vi "Untitled 1.vi"() -> ()   [LabVIEW 2016]
uses:
  support/Message Queue/Message Queue.lvlib
  support/Message Queue/Enqueue Message (Single).vi
  controls/UI State.ctl
  Settings/Settings.lvlib
  support/User Event - Stop/User Event - Stop.lvlib
  <vilib>/Utility/error.llb/Error Cluster From Error Code.vi
  <vilib>/ErrorRing/Error Ring.xnode
panel:
  in  "PZTY+":bool
  in  "PZTX-":bool
  in  "PZTX+":bool
  in  "PZTY-":bool
  in  "PZTZ-":bool
  in  "PZTZ+":bool
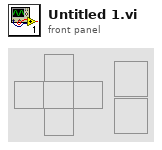
[diagram p1: front panel]
types:
  T1 = typedef "UI State.ctl" = enum16{"Idle", "Acquiring", "Acquiring Stopped", "Logging", "Logging Stopped"}
  T2 = typedef "Settings.lvlib/Settings.ctl" = cluster{"Hardware Configuration":T3, "Logging Configuration":T4, "PZT Configuration ":T5}
  T3 = typedef "Acquisition.lvlib/Hardware Configuration.ctl" = cluster{"DAQmx Input":tag, "Max Input":dbl, "Min Input":dbl, "Sample Rate":dbl, "DAQmx Task":refnum<k21>}
  T4 = typedef "Logging.lvlib/Logging Configuration.ctl" = cluster{"Log File Base Path":path, "TDMS File Reference":refnum<k34>, "Channel names":string[], "Author":string, "Description":string}
  T5 = typedef "PZT_Control.ctl" = cluster{"DAQmx Output":tag, "PZTX":dbl, "PZTY":dbl, "PZTZ":dbl, "Waveform Type":enum16{"Sine Wave", "Triangle Wave", "Square Wave", "Sawtooth Wave"}, "PZT_Amp":dbl, "PZT_Freq":dbl, "PZT_Phase":dbl}
  T6 = cluster{"Hardware Configuration":T3, "Logging Configuration":cluster{"Log File Base Path":path, "TDMS File Reference":refnum<k34>, "Channel names":string[], "Author":string, "Description":string}, "PZT Configuration ":T5}
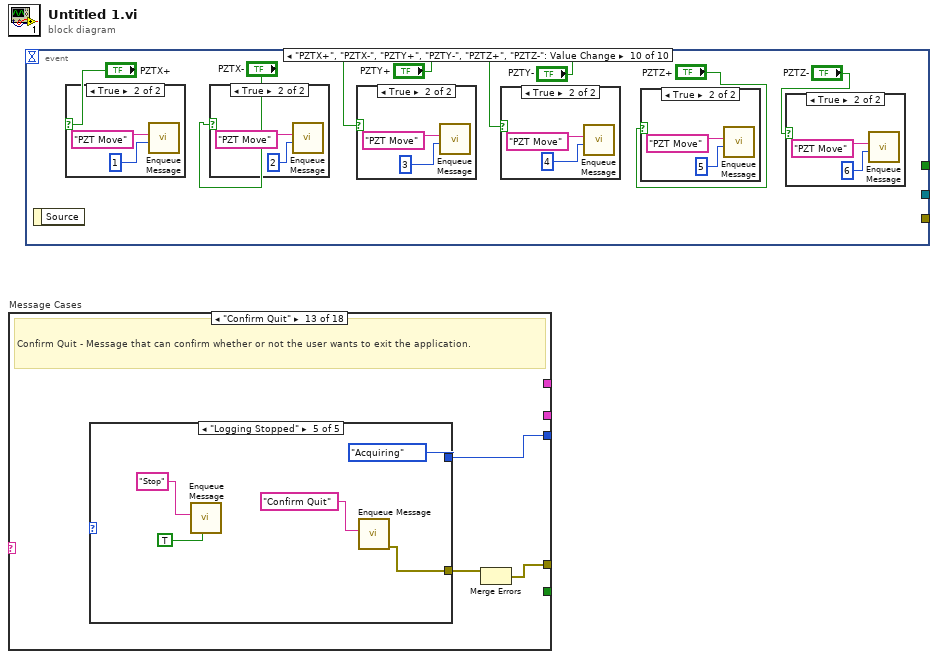
[diagram p0: block diagram]
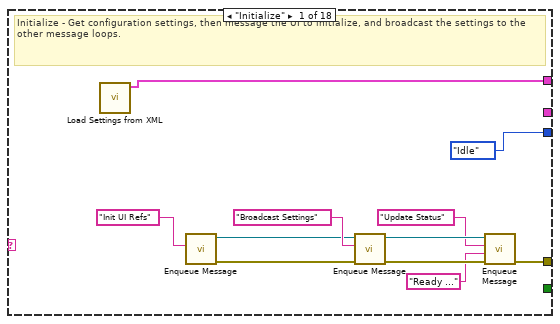
[diagram p2: hidden frame]
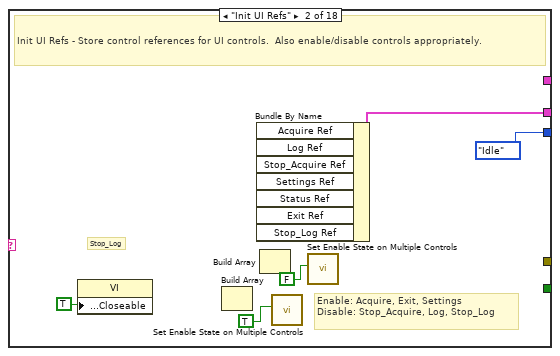
[diagram p3: hidden frame]
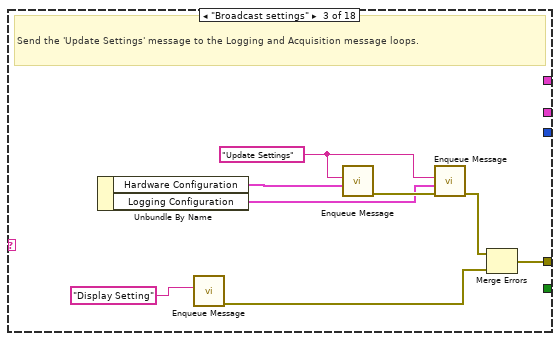
[diagram p4: hidden frame]
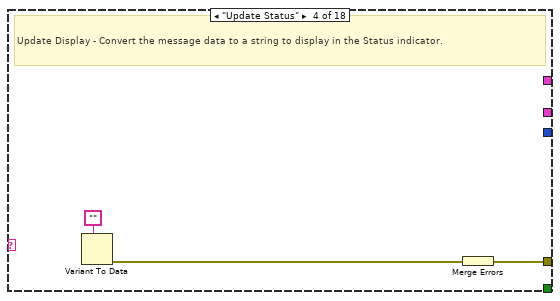
[diagram p5: hidden frame]
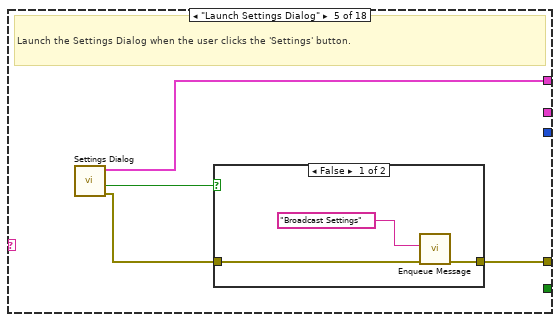
[diagram p6: hidden frame]
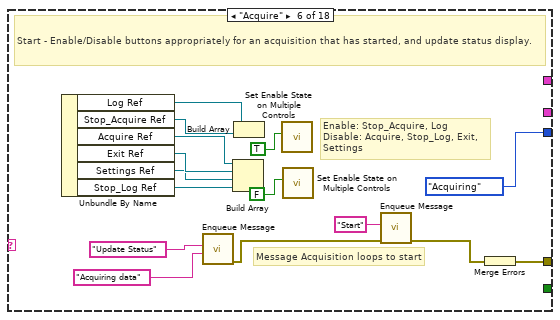
[diagram p8: hidden frame]
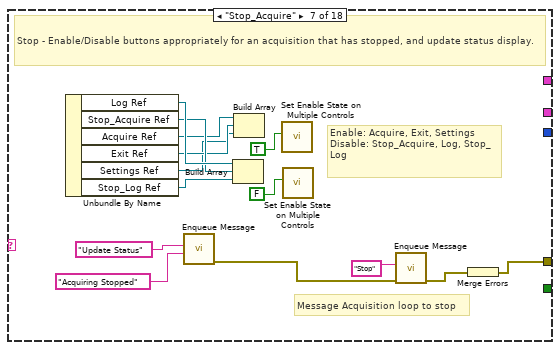
[diagram p9: hidden frame]
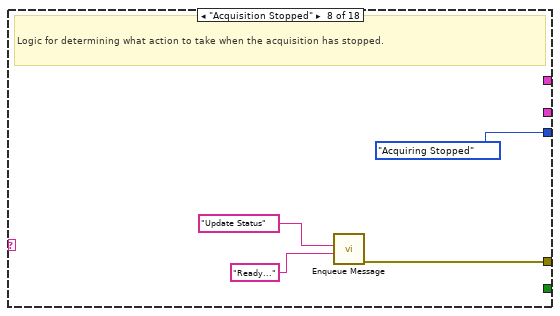
[diagram p10: hidden frame]
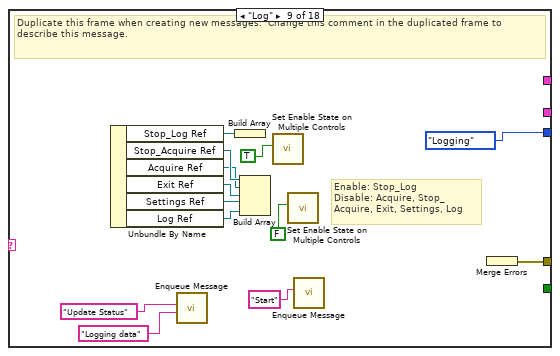
[diagram p11: hidden frame]
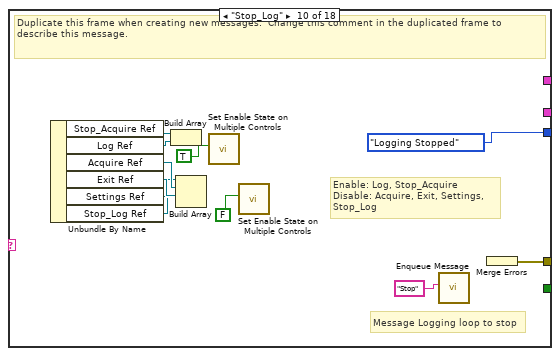
[diagram p12: hidden frame]
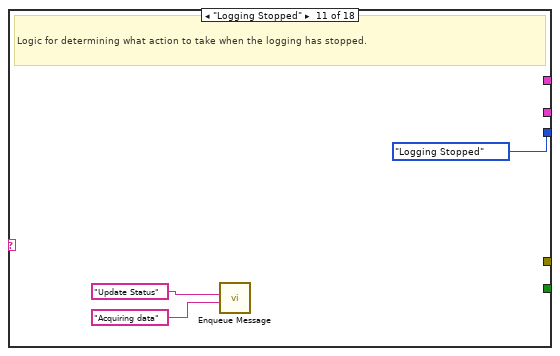
[diagram p13: hidden frame]
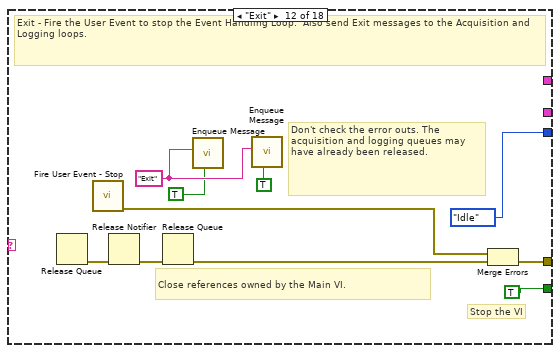
[diagram p14: hidden frame]
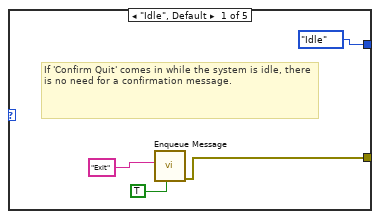
[diagram p15: hidden frame]
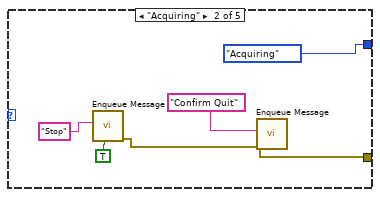
[diagram p16: hidden frame]
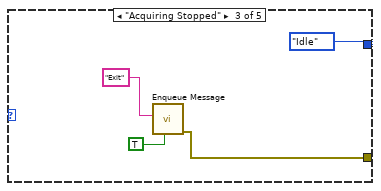
[diagram p17: hidden frame]
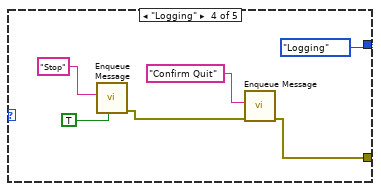
[diagram p18: hidden frame]
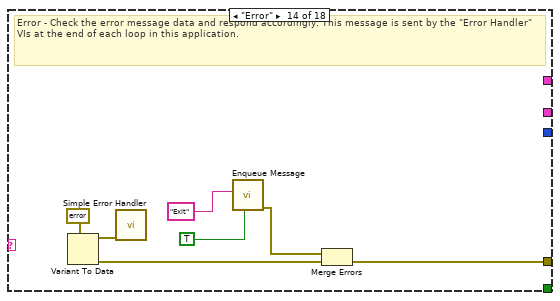
[diagram p19: hidden frame]
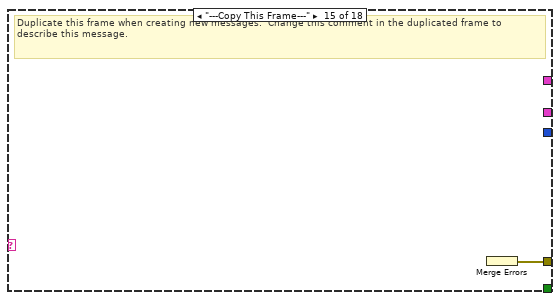
[diagram p20: hidden frame]
diagram:
  n1 = case "Message Cases" shown="\"Confirm Quit\"" {
    selector: _ -> [_ _ _ _ _ _ _ _ _ _ _ _ _ _ _ _ _ w145]
    tunnel: [w9 _ w24 w27 w29 w50 w64 w67 w81 w92 _ w104 w107 w134 w141 _ w144 w146] -> _
    tunnel: [_ _ _ _ _ _ _ _ _ _ _ TRUE _ _ _ _ _ _] -> _
    tunnel: [_ w16 _ _ _ _ _ _ _ _ _ _ _ _ _ _ _ _] -> _
    tunnel: [UI_State."Idle" ("UI State") UI_State."Idle" ("UI State") _ _ _ UI_State."Acquiring" ("UI State") _ UI_State."Acquiring Stopped" ("UI State") UI_State."Logging" ("UI State") UI_State."Logging Stopped" ("UI State") UI_State."Logging Stopped" ("UI State") UI_State."Idle" ("UI State") w108 _ _ _ _ _] -> _
    tunnel: [w1 _ _ _ w28 _ _ _ _ _ _ _ _ _ _ _ _ _] -> _
    frame "Initialize" {
      # "Initialize - Get configuration settings, then message the UI to initialize, and broadcast the settings to the other message loops."
      n2 = call "Load Settings from XML.vi"() -> ("Settings out"=w1:T2)  [unwired: 10 in, 1 out]
      n3 = call-poly "Enqueue Message.vi"("Message"="Init UI Refs") -> ("error out"=w3:errorcluster, "dup Message Queue"=w4:refnum<queue>)  [unwired: 9 in]
      n4 = call-poly "Enqueue Message.vi"("error in (no error)"=w3, "Message"="Broadcast Settings", "Message Queue"=w4) -> ("error out"=w11:errorcluster, "dup Message Queue"=w10:refnum<queue>)  [unwired: 7 in]
      n5 = call-poly "Enqueue Message.vi"("error in (no error)"=w11, "Message Data"="Ready ..." ("Ready..."), "Message"="Update Status", "Message Queue"=w10) -> ("error out"=w9:errorcluster)  [unwired: 6 in, 1 out]
    }
    frame "Init UI Refs" {
      # "Stop_Log"
      # "Enable: Acquire, Exit, Settings\nDisable: Stop_Acquire, Log, Stop_Log"
      # "Init UI Refs - Store control references for UI controls.  Also enable/disable controls appropriately."
      n6 = property class="VI"("Front Panel.Closeable"=TRUE ("Front Panel Window:Closeable")) -> ()  [unwired: 2 in, 2 out]
      n7 = Build Array() -> ()  [unwired: 3 in, 1 out]
      n8 = Bundle By Name() -> (w16:cluster{})  [unwired: 8 in]
      n9 = Build Array() -> ()  [unwired: 3 in, 1 out]
      n10 = call "Set Enable State on Multiple Controls.vi"("Enable?"=TRUE) -> ()  [unwired: 11 in]
      n11 = call "Set Enable State on Multiple Controls.vi"("Enable?"=FALSE) -> ()  [unwired: 11 in]
    }
    frame "Broadcast settings" {
      w19 = "Update Settings" ("Message")
      # "Send the 'Update Settings' message to the Logging and Acquisition message loops."
      n12 = Unbundle By Name() -> ("Hardware Configuration"=w22:T3, "Logging Configuration"=w21:T4)  [unwired: 1 in]
      n13 = call-poly "Enqueue Message.vi"("Message"="Display Setting") -> ("error out"=w17:errorcluster)  [unwired: 9 in, 1 out]
      n14 = call-poly "Enqueue Message.vi"("Message Data"=w22, "Message"=w19) -> ("error out"=w23:errorcluster)  [unwired: 8 in, 1 out]
      n15 = call-poly "Enqueue Message.vi"("error in (no error)"=w23, "Message Data"=w21, "Message"=w19) -> ("error out"=w20:errorcluster)  [unwired: 7 in, 1 out]
      n16 = Merge Errors(w20, w17) -> (w24:errorcluster)  [unwired: 1 in]
    }
    frame "Update Status" {
      # "Update Display - Convert the message data to a string to display in the Status indicator."
      n17 = Variant To Data(type="") -> (error out=w25:errorcluster)  [unwired: 2 in, 1 out]
      n18 = Merge Errors(w25) -> (w27:errorcluster)
    }
    frame "Launch Settings Dialog" {
      # "Launch the Settings Dialog when the user clicks the 'Settings' button."
      n19 = call "Settings Dialog.vi"() -> ("error out"=w30:errorcluster, "Cancelled?"=w31:bool, "Settings out"=w28:T6)  [unwired: 8 in, 1 out]
      n20 = case shown="False" w31 {
        tunnel: w30 -> [w34 w35]
        tunnel: [w33 w35] -> w29
        frame False {
          n21 = call-poly "Enqueue Message.vi"("error in (no error)"=w34, "Message"="Broadcast Settings") -> ("error out"=w33:errorcluster)  [unwired: 8 in, 1 out]
        }
        frame True {
        }
      }
    }
    frame "Acquire" {
      # "Message Acquisition loops to start"
      # "Enable: Stop_Acquire, Log\nDisable: Acquire, Stop_Log, Exit, Settings"
      # "Start - Enable/Disable buttons appropriately for an acquisition that has started, and update status display."
      n22 = Unbundle By Name() -> ("Log Ref"=w39:refnum<vi>, "Stop_Acquire Ref"=w40:refnum<vi>, "Acquire Ref"=w45:refnum<vi>, "Exit Ref"=w44:refnum<vi>, "Settings Ref"=w43:refnum<vi>, "Stop_Log Ref"=w36:refnum<vi>)  [unwired: 1 in]
      n23 = call-poly "Enqueue Message.vi"("Message Data"="Acquiring data" ("Waiting for trigger"), "Message"="Update Status") -> ("error out"=w37:errorcluster)  [unwired: 8 in, 1 out]
      n24 = Build Array(w45, w44, w43, w36) -> ()  [unwired: 1 out]
      n25 = Build Array(w39, w40) -> ()  [unwired: 1 out]
      n26 = call "Set Enable State on Multiple Controls.vi"("Enable?"=TRUE) -> ()  [unwired: 11 in]
      n27 = call "Set Enable State on Multiple Controls.vi"("Enable?"=FALSE) -> ()  [unwired: 11 in]
      n28 = call-poly "Enqueue Message.vi"("error in (no error)"=w37, "Message"="Start") -> ("error out"=w42:errorcluster)  [unwired: 8 in, 1 out]
      n29 = Merge Errors(w42) -> (w50:errorcluster)
    }
    frame "Stop_Acquire" {
      # "Message Acquisition loop to stop"
      # "Enable: Acquire, Exit, Settings\nDisable: Stop_Acquire, Log, Stop_Log"
      # "Stop - Enable/Disable buttons appropriately for an acquisition that has stopped, and update status display."
      n30 = Unbundle By Name() -> ("Log Ref"=w57:refnum<vi>, "Stop_Acquire Ref"=w56:refnum<vi>, "Acquire Ref"=w55:refnum<vi>, "Exit Ref"=w54:refnum<vi>, "Settings Ref"=w53:refnum<vi>, "Stop_Log Ref"=w52:refnum<vi>)  [unwired: 1 in]
      n31 = call-poly "Enqueue Message.vi"("Message Data"="Acquiring Stopped" ("Ready..."), "Message"="Update Status") -> ("error out"=w51:errorcluster)  [unwired: 8 in, 1 out]
      n32 = Build Array(w57, w56, w52) -> ()  [unwired: 1 out]
      n33 = Build Array(w55, w54, w53) -> ()  [unwired: 1 out]
      n34 = call "Set Enable State on Multiple Controls.vi"("Enable?"=TRUE) -> ()  [unwired: 11 in]
      n35 = call "Set Enable State on Multiple Controls.vi"("Enable?"=FALSE) -> ()  [unwired: 11 in]
      n36 = call-poly "Enqueue Message.vi"("error in (no error)"=w51, "Message"="Stop") -> ("error out"=w59:errorcluster)  [unwired: 8 in, 1 out]
      n37 = Merge Errors(w59) -> (w64:errorcluster)
    }
    frame "Acquisition Stopped" {
      # "Logic for determining what action to take when the acquisition has stopped."
      n38 = call-poly "Enqueue Message.vi"("Message Data"="Ready..." ("Message"), "Message"="Update Status") -> ("error out"=w67:errorcluster)  [unwired: 8 in, 1 out]
    }
    frame "Log" {
      # "Enable: Stop_Log\nDisable: Acquire, Stop_Acquire, Exit, Settings, Log"
      # "Duplicate this frame when creating new messages.  Change this comment in the duplicated frame to describe this message."
      n39 = Unbundle By Name() -> ("Stop_Log Ref"=w75:refnum<vi>, "Stop_Acquire Ref"=w74:refnum<vi>, "Acquire Ref"=w73:refnum<vi>, "Exit Ref"=w72:refnum<vi>, "Settings Ref"=w71:refnum<vi>, "Log Ref"=w70:refnum<vi>)  [unwired: 1 in]
      n40 = call-poly "Enqueue Message.vi"("Message Data"="Logging data" ("Ready..."), "Message"="Update Status") -> ()  [unwired: 8 in, 2 out]
      n41 = Build Array(w75) -> ()  [unwired: 1 out]
      n42 = Build Array(w74, w73, w72, w71, w70) -> ()  [unwired: 1 out]
      n43 = call "Set Enable State on Multiple Controls.vi"("Enable?"=TRUE) -> ()  [unwired: 11 in]
      n44 = call "Set Enable State on Multiple Controls.vi"("Enable?"=FALSE) -> ()  [unwired: 11 in]
      n45 = call-poly "Enqueue Message.vi"("Message"="Start") -> ()  [unwired: 9 in, 2 out]
      n46 = Merge Errors() -> (w81:errorcluster)  [unwired: 1 in]
    }
    frame "Stop_Log" {
      # "Message Logging loop to stop"
      # "Enable: Log, Stop_Acquire\nDisable: Acquire, Exit, Settings, Stop_Log"
      # "Duplicate this frame when creating new messages.  Change this comment in the duplicated frame to describe this message."
      n47 = Unbundle By Name() -> ("Stop_Acquire Ref"=w88:refnum<vi>, "Log Ref"=w84:refnum<vi>, "Acquire Ref"=w87:refnum<vi>, "Exit Ref"=w86:refnum<vi>, "Settings Ref"=w85:refnum<vi>, "Stop_Log Ref"=w83:refnum<vi>)  [unwired: 1 in]
      n48 = Build Array(w88, w84) -> ()  [unwired: 1 out]
      n49 = Build Array(w83, w87, w86, w85) -> ()  [unwired: 1 out]
      n50 = call "Set Enable State on Multiple Controls.vi"("Enable?"=TRUE) -> ()  [unwired: 11 in]
      n51 = call "Set Enable State on Multiple Controls.vi"("Enable?"=FALSE) -> ()  [unwired: 11 in]
      n52 = call-poly "Enqueue Message.vi"("Message"="Stop") -> ()  [unwired: 9 in, 2 out]
      n53 = Merge Errors() -> (w92:errorcluster)  [unwired: 1 in]
    }
    frame "Logging Stopped" {
      # "Logic for determining what action to take when the logging has stopped."
      n54 = call-poly "Enqueue Message.vi"("Message Data"="Acquiring data" ("Ready..."), "Message"="Update Status") -> ()  [unwired: 8 in, 2 out]
    }
    frame "Exit" {
      w102 = "Exit" ("Message")
      # "Don't check the error outs. The acquisition and logging queues may have already been released."
      # "Close references owned by the Main VI."
      # "Stop the VI"
      # "Exit - Fire the User Event to stop the Event Handling Loop.  Also send Exit messages to the Acquisition and Logging loops."
      n55 = Release Queue() -> (error out=w101:errorcluster)  [unwired: 3 in, 2 out]
      n56 = call "Fire User Event - Stop.vi"() -> ("error out"=w103:errorcluster)  [unwired: 11 in]
      n57 = Release Notifier(error in (no error)=w101) -> (error out=w100:errorcluster)  [unwired: 2 in, 2 out]
      n58 = Release Queue(error in (no error)=w100) -> (error out=w99:errorcluster)  [unwired: 2 in, 2 out]
      n59 = call-poly "Enqueue Message.vi"("Priority Message? (F)"=TRUE, "Message"=w102) -> ()  [unwired: 8 in, 2 out]
      n60 = call-poly "Enqueue Message.vi"("Priority Message? (F)"=TRUE, "Message"=w102) -> ()  [unwired: 8 in, 2 out]
      n61 = Merge Errors(w103, w99) -> (w104:errorcluster)
    }
    frame "Confirm Quit" {
      # "Confirm Quit - Message that can confirm whether or not the user wants to exit the application."
      n62 = case shown="\"Logging Stopped\"" {
        selector: _ -> [_ _ _ _ _]
        tunnel: [w110 w114 w119 w123 w129] -> w106
        tunnel: [UI_State."Idle" ("UI State") UI_State."Acquiring" ("UI State") UI_State."Idle" ("UI State") UI_State."Logging" ("UI State") UI_State."Acquiring" ("UI State")] -> w108
        frame "Idle", Default {
          # "If 'Confirm Quit' comes in while the system is idle, there is no need for a confirmation message."
          n63 = call-poly "Enqueue Message.vi"("Priority Message? (F)"=TRUE, "Message"="Exit") -> ("error out"=w110:errorcluster)  [unwired: 8 in, 1 out]
        }
        frame "Acquiring" {
          n64 = call-poly "Enqueue Message.vi"("Priority Message? (F)"=TRUE, "Message"="Stop") -> ("error out"=w115:errorcluster)  [unwired: 8 in, 1 out]
          n65 = call-poly "Enqueue Message.vi"("error in (no error)"=w115, "Message"="Confirm Quit") -> ("error out"=w114:errorcluster)  [unwired: 8 in, 1 out]
        }
        frame "Acquiring Stopped" {
          n66 = call-poly "Enqueue Message.vi"("Priority Message? (F)"=TRUE, "Message"="Exit") -> ("error out"=w119:errorcluster)  [unwired: 8 in, 1 out]
        }
        frame "Logging" {
          n67 = call-poly "Enqueue Message.vi"("Priority Message? (F)"=TRUE, "Message"="Stop") -> ("error out"=w124:errorcluster)  [unwired: 8 in, 1 out]
          n68 = call-poly "Enqueue Message.vi"("error in (no error)"=w124, "Message"="Confirm Quit") -> ("error out"=w123:errorcluster)  [unwired: 8 in, 1 out]
        }
        frame "Logging Stopped" {
          n69 = call-poly "Enqueue Message.vi"("Priority Message? (F)"=TRUE, "Message"="Stop") -> ()  [unwired: 8 in, 2 out]
          n70 = call-poly "Enqueue Message.vi"("Message"="Confirm Quit") -> ("error out"=w129:errorcluster)  [unwired: 9 in, 1 out]
        }
      }
      n71 = Merge Errors(w106) -> (w107:errorcluster)  [unwired: 1 in]
    }
    frame "Error" {
      # "Error - Check the error message data and respond accordingly. This message is sent by the \"Error Handler\" VIs at the end of each loop in this application."
      n72 = Variant To Data(type=errorcluster {"status"=FALSE, "code"=0, "source"=""} ("error out")) -> (data=w139:errorcluster, error out=w136:errorcluster)  [unwired: 2 in]
      n73 = call <vilib>:"Simple Error Handler.vi"("error in (no error)"=w139) -> ()  [unwired: 4 in, 5 out]
      n74 = call-poly "Enqueue Message.vi"("Priority Message? (F)"=TRUE, "Message"="Exit") -> ("error out"=w135:errorcluster)  [unwired: 8 in, 1 out]
      n75 = Merge Errors(w135, w136) -> (w134:errorcluster)
    }
    frame "---Copy This Frame---" {
      # "Duplicate this frame when creating new messages.  Change this comment in the duplicated frame to describe this message."
      n76 = Merge Errors() -> (w141:errorcluster)  [unwired: 1 in]
    }
    frame "PZT Move" {
      n77 = Variant To Data(type=0 ("Message")) -> (data=w142:i32)  [unwired: 2 in, 1 out]
      n78 = case shown="4" w142 {
        frame Default {
          n79 = local read item#-1() -> ()  [unwired: 1 in]
        }
        frame 1 {
        }
        frame 2 {
          n80 = local read item#-1() -> ()  [unwired: 1 in]
        }
        frame 3 {
          n81 = local read item#-1() -> ()  [unwired: 1 in]
        }
        frame 4 {
          n82 = local read item#-1() -> ()  [unwired: 1 in]
        }
        frame 5 {
          n83 = local read item#-1() -> ()  [unwired: 1 in]
        }
        frame 6 {
          n84 = local read item#-1() -> ()  [unwired: 1 in]
        }
      }
    }
    frame "Display Setting" {
      # "Duplicate this frame when creating new messages.  Change this comment in the duplicated frame to describe this message."
      n85 = Unbundle By Name() -> ()  [unwired: 1 in, 3 out]
      n86 = Merge Errors() -> (w144:errorcluster)  [unwired: 1 in]
    }
    frame Default {
      # "'Default' case only runs if there is a message that isn't defined in any of the other cases.  Output a programming error."
      n87 = xnode "Error Ring"("parameter 0"=w145) -> ("error out"=w146:errorcluster)
    }
  }
  n88 = event shown="[9] \"PZTX+\", \"PZTX-\", \"PZTY+\", \"PZTY-\", \"PZTZ+\", \"PZTZ-\": Value Change" {
    selector: _ -> [_ _ _ _ _ _ _ _ _ _]
    dyn-events: _ -> [_ _ _ _ _ _ _ _ _ _]
    timeout: _ -> [_ _ _ _ _ _ _ _ _ _]
    tunnel: [_ _ _ _ _ _ _ _ TRUE ("Discard?") _] -> _
    tunnel: [w156 w159 w161 _ w166 w171 _ w172 _ _] -> _
    tunnel: [w154 w157 w160 w164 w165 w168 _ w173 _ _] -> _
    event #0 (no event record) {
      n89 = event-data() -> ()  [unwired: 1 in, 1 out]
      n90 = call-poly "Enqueue Message.vi"("Message"="Launch Settings Dialog") -> ("error out"=w156:errorcluster, "dup Message Queue"=w154:refnum<queue>)  [unwired: 9 in]
    }
    event #1 (no event record) {
      n91 = event-data() -> ()  [unwired: 1 in, 1 out]
      n92 = call-poly "Enqueue Message.vi"("Message"="Acquire") -> ("error out"=w159:errorcluster, "dup Message Queue"=w157:refnum<queue>)  [unwired: 9 in]
    }
    event #2 (no event record) {
      n93 = event-data() -> ()  [unwired: 1 in, 1 out]
      n94 = call-poly "Enqueue Message.vi"("Message"="Stop_Acquire") -> ("error out"=w161:errorcluster, "dup Message Queue"=w160:refnum<queue>)  [unwired: 9 in]
    }
    event #3 (no event record) {
      n95 = event-data() -> ()  [unwired: 1 in, 1 out]
      n96 = call-poly "Enqueue Message.vi"("Message"="Log") -> ("dup Message Queue"=w164:refnum<queue>)  [unwired: 9 in, 1 out]
    }
    event #4 (no event record) {
      n97 = event-data() -> ()  [unwired: 1 in, 1 out]
      n98 = call-poly "Enqueue Message.vi"("Message"="Stop_Log") -> ("error out"=w166:errorcluster, "dup Message Queue"=w165:refnum<queue>)  [unwired: 9 in]
    }
    event Panel Close {
      w169 = TRUE  # Priority Message
      # "The UI Message Loop handles sending the Exit message to other loops."
      n99 = event-data() -> ()  [unwired: 1 in, 1 out]
      n100 = call-poly "Enqueue Message.vi"("Priority Message? (F)"=w169, "Message"="Exit") -> ("error out"=w171:errorcluster, "dup Message Queue"=w168:refnum<queue>)  [unwired: 8 in]
    }
    event Application Instance Close {
      n101 = event-data() -> ()  [unwired: 1 in, 1 out]
    }
    event Panel Close? {
      # "Send the 'Confirm Quit' message if the user closes the panel of the VI. Discard the event so the 'Confirm Quit' message has a chance to run."
      n102 = event-data() -> ()  [unwired: 1 in, 1 out]
      n103 = call-poly "Enqueue Message.vi"("Priority Message? (F)"=TRUE, "Message"="Confirm Quit") -> ("error out"=w172:errorcluster, "dup Message Queue"=w173:refnum<queue>)  [unwired: 8 in]
      n104 = event-data("Discard?"=TRUE) -> ()  [unwired: 1 in, 1 out]
    }
    event User Event {
      (unwired) "Exit" ("Exit String")
      # "The Message Handling Loop processed an \"Exit\" message, which fired this event to stop the Event Handling Loop."
      n105 = event-data() -> ()  [unwired: 1 in, 1 out]
      n106 = local read item#-1() -> ()  [unwired: 1 in]
    }
    event "PZTX+", "PZTX-", "PZTY+", "PZTY-", "PZTZ+", "PZTZ-": Value Change {
      n107 = event-data() -> ()  [unwired: 1 in, 1 out]
      n108 = case shown="True" "PZTX+" {
        frame False {
        }
        frame True {
          n109 = call-poly "Enqueue Message.vi"("Message Data"=1 ("Message"), "Message"="PZT Move") -> ()  [unwired: 8 in, 2 out]
        }
      }
      n110 = case shown="True" "PZTX-" {
        frame False {
        }
        frame True {
          n111 = call-poly "Enqueue Message.vi"("Message Data"=2 ("Message"), "Message"="PZT Move") -> ()  [unwired: 8 in, 2 out]
        }
      }
      n112 = case shown="True" "PZTY+" {
        frame False {
        }
        frame True {
          n113 = call-poly "Enqueue Message.vi"("Message Data"=3 ("Message"), "Message"="PZT Move") -> ()  [unwired: 8 in, 2 out]
        }
      }
      n114 = case shown="True" "PZTY-" {
        frame False {
        }
        frame True {
          n115 = call-poly "Enqueue Message.vi"("Message Data"=4 ("Message"), "Message"="PZT Move") -> ()  [unwired: 8 in, 2 out]
        }
      }
      n116 = case shown="True" "PZTZ+" {
        frame False {
        }
        frame True {
          n117 = call-poly "Enqueue Message.vi"("Message Data"=5 ("Message"), "Message"="PZT Move") -> ()  [unwired: 8 in, 2 out]
        }
      }
      n118 = case shown="True" "PZTZ-" {
        frame False {
        }
        frame True {
          n119 = call-poly "Enqueue Message.vi"("Message Data"=6 ("Message"), "Message"="PZT Move") -> ()  [unwired: 8 in, 2 out]
        }
      }
    }
  }
